vi "Destroy.vi"(0 "reference in":refnum<class "AI.lvclass">, 5 "error in (no error)":errorcluster) -> (14 "reference out":refnum<class "AI.lvclass">, 19 "error out":errorcluster)   [LabVIEW 2017, in "AI.lvclass"]
uses:
  AI.lvclass
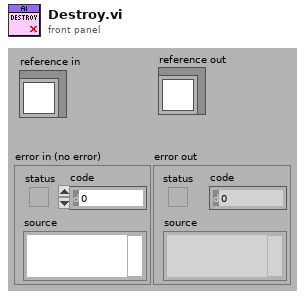
[diagram p1: front panel]
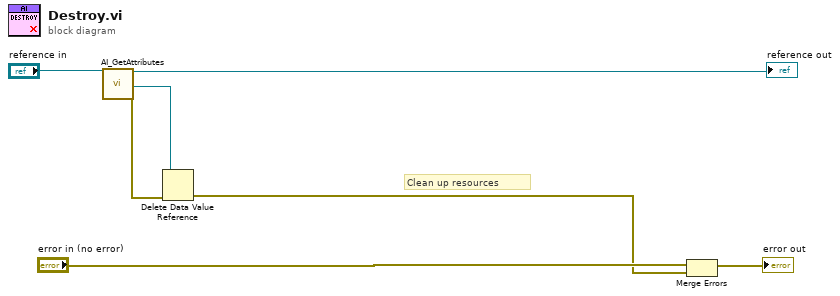
[diagram p0: block diagram]
diagram:
  # "Clean up resources"
  n1 = call "AI_GetAttributes.vi"("reference in"="reference in") -> ("reference out"=→"reference out":refnum<class "AI.lvclass">, "DataRef"=w1:refnum<data-value>, "error out"=w4:errorcluster)  [unwired: 15 in, 1 out]
  n2 = Delete Data Value Reference(data value reference=w1, error in=w4) -> (error out=w2:errorcluster)  [unwired: 1 out]
  n3 = Merge Errors("error in (no error)", w2) -> (→"error out":errorcluster)
